vi "AutonomousMode.vi"() -> ()   [LabVIEW 2016]
panel:
  out "ROS NOTSTOPP!!! -> wird über am:0 entschärft":bool
  out "If true -> Strassenparameter; if false -> Hebebühne":bool
  out "Run Regler=Autonomous Mode":bool
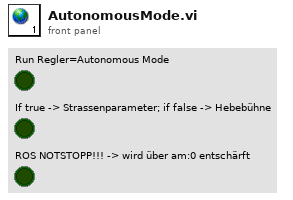
[diagram p1: front panel]
diagram:
